vi "Feeder Move Elevator.vi"(8 "error in (no error)":errorcluster, 11 "Action":enum16{"Drop", "Lift"}(ring)=enum."Lift") -> (0 "error out":errorcluster)   [LabVIEW 2014]
uses:
  Main/Robot Global Data.vi
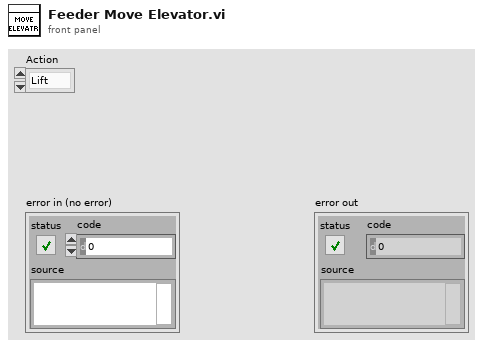
[diagram p1: front panel]
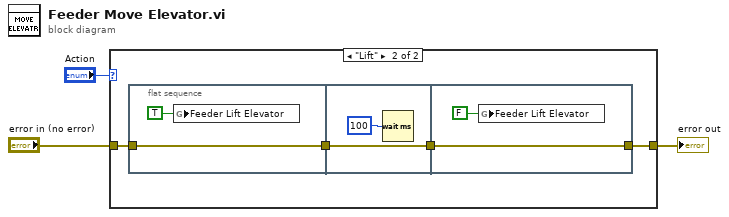
[diagram p0: block diagram]
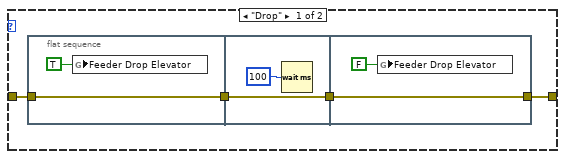
[diagram p2: hidden frame]
diagram:
  n1 = case shown="\"Lift\"" "Action" {
    tunnel: "error in (no error)" -> [w6 w17]
    tunnel: [w4 w14] -> w1
    frame "Drop" {
      n2 = flat-sequence {
        tunnel: [w8] -> w7
        tunnel: w6 -> [w8]
        tunnel: w7 -> [w10]
        tunnel: [w10] -> w5
        tunnel: [w12] -> w4
        tunnel: w5 -> [w12]
        frame #0 {
          n3 = global write "Robot Global Data.vi" "Feeder Drop Elevator"(TRUE ("Feeder Drop Elevator")) -> ()
        }
        frame #1 {
          n4 = Wait (ms)(milliseconds to wait=u32 100) -> ()  [unwired: 1 out]
        }
        frame #2 {
          n5 = global write "Robot Global Data.vi" "Feeder Drop Elevator"(FALSE ("Feeder Drop Elevator")) -> ()
        }
      }
    }
    frame "Lift" {
      n6 = flat-sequence {
        tunnel: w17 -> [w18]
        tunnel: [w18] -> w15
        tunnel: [w20] -> w16
        tunnel: w15 -> [w20]
        tunnel: [w22] -> w14
        tunnel: w16 -> [w22]
        frame #0 {
          n7 = global write "Robot Global Data.vi" "Feeder Lift Elevator"(TRUE ("Feeder Drop Elevator")) -> ()
        }
        frame #1 {
          n8 = Wait (ms)(milliseconds to wait=u32 100) -> ()  [unwired: 1 out]
        }
        frame #2 {
          n9 = global write "Robot Global Data.vi" "Feeder Lift Elevator"(FALSE ("Feeder Drop Elevator")) -> ()
        }
      }
    }
  }
  "error out" <- w1
